vi "get_serv_msgs.vi"() -> ()   [LabVIEW 2010]
uses:
  <vilib>/httpClient/LabVIEWHTTPClient.lvlib
panel:
  out "date/time string":string
  in  "Tab Control":enum32{"Page 1", "Page 2"}(tab)
  out "body":string
  out "Table Control":string[][](table)
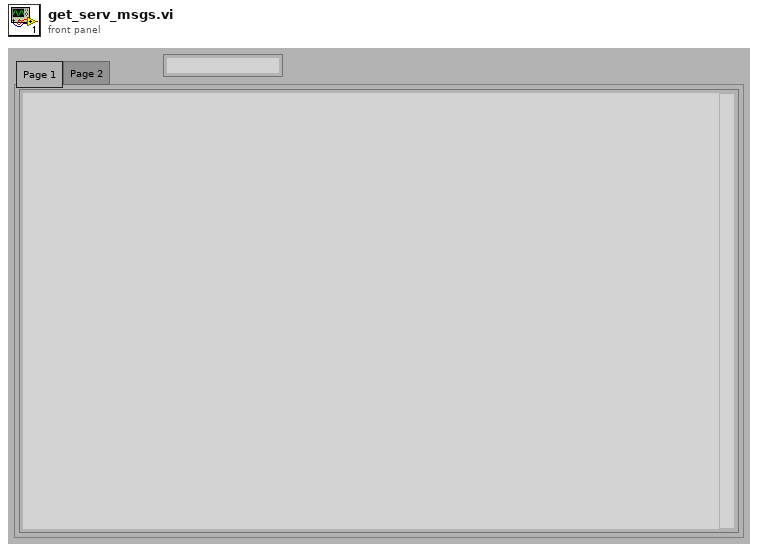
[diagram p1: front panel]
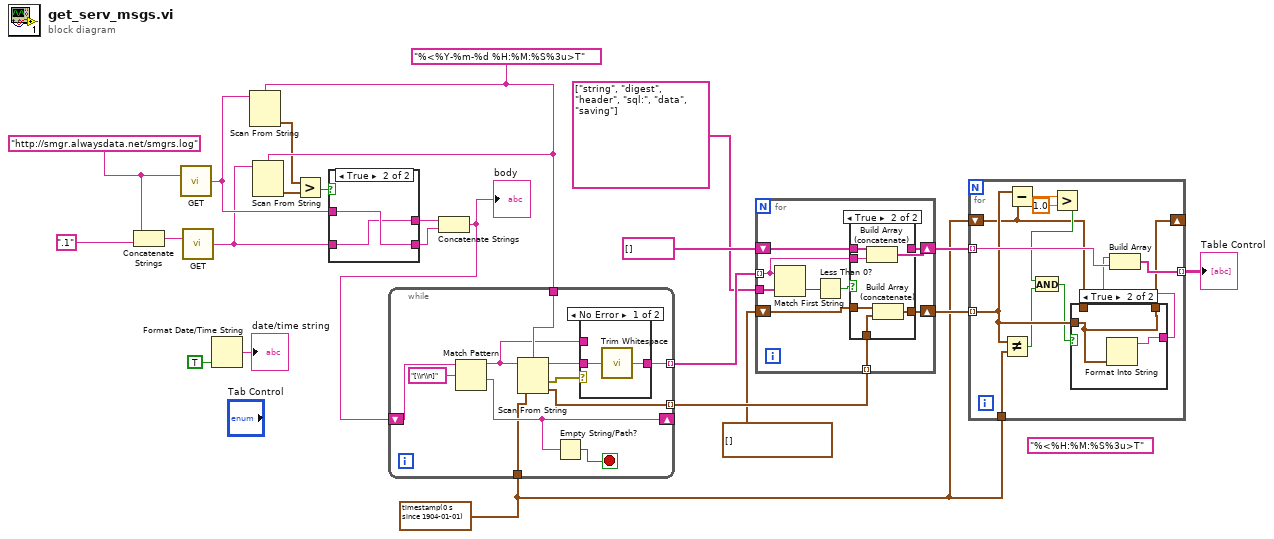
[diagram p0: block diagram]
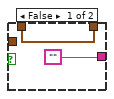
[diagram p2: hidden frame]
diagram:
  (unwired) "%<%H:%M:%S%3u>T" ("format string")
  w3 = timestamp(0 s since 1904-01-01) ("default value 1")
  w15 = "%<%Y-%m-%d %H:%M:%S%3u>T" ("format string")
  w16 = "http://smgr.alwaysdata.net/smgrs.log" ("URL")
  n1 = Concatenate Strings(w16, ".1" ("string")) -> (w19:string)
  n2 = call <vilib>:"GET.vi"("URL"=w16) -> ("body"=w10:string)  [unwired: 11 in, 3 out]
  n3 = call <vilib>:"GET.vi"("URL"=w19) -> ("body"=w9:string)  [unwired: 11 in, 3 out]
  n4 = Format Date/Time String(UTC format=TRUE) -> (date/time string=→"date/time string":string)  [unwired: 2 in]
  n5 = Scan From String(format string=w15, input string=w10) -> (output 1=w14:timestamp)  [unwired: 3 in, 3 out]
  n6 = Scan From String(format string=w15, input string=w9) -> (output 1=w13:timestamp)  [unwired: 3 in, 3 out]
  n7 = Greater?(x=w14, y=w13) -> (0:w12:bool)
  n8 = case shown="True" w12 {
    tunnel: w10 -> [w24 w27]
    tunnel: w9 -> [w25 w26]
    tunnel: [w25 w27] -> w8
    tunnel: [w24 w26] -> w7
    frame False {
    }
    frame True {
    }
  }
  n9 = Concatenate Strings(w7, w8) -> (w11:string)
  "body" <- w11
  n10 = while {
    shift-right: [w35] -> _
    shift-left: w11 -> [w37]
    tunnel: [w31] -> w23 mode=indexing
    tunnel: w15 -> [w34]
    tunnel: [w29] -> w18 mode=indexing
    tunnel: w3 -> [w28]
    stop <- w36 stop-if-true
    n11 = Match Pattern(string=w37, regular expression="[\\r\\n]") -> (before substring=w30:string, after substring=w35:string)  [unwired: 1 in, 2 out]
    n12 = Scan From String(format string=w34, input string=w30, default 1=w28) -> (remaining string=w32:string, error out=w33:errorcluster, output 1=w29:timestamp)  [unwired: 2 in, 1 out]
    n13 = Empty String/Path?(string/path=w35) -> (empty?=w36:bool)
    n14 = case shown="No Error" w33 {
      tunnel: [w39 w41] -> w31
      tunnel: w32 -> [w40 _]
      tunnel: w30 -> [_ w41]
      frame No Error {
        n15 = call <vilib>:"Trim Whitespace.vi"("string"=w40) -> ("trimmed string"=w39:string)  [unwired: 1 in]
      }
      frame Error {
      }
    }
  }
  n16 = for {
    tunnel: w23 -> [w48] mode=indexing
    shift-right: [w47] -> w5
    shift-left: string[] [] -> [w46]
    tunnel: string[] ["string", "digest", "header", "sql:", "data", "saving"] -> [w45]
    tunnel: w18 -> [w44] mode=indexing
    shift-right: [w43] -> w6
    shift-left: timestamp[] [] -> [w42]
    n17 = Match First String(2:w45, 3:w48) -> (0:w50:i32)  [unwired: 1 out]
    n18 = Less Than 0?(x=w50) -> (x < 0?=w49:bool)
    n19 = case shown="True" w49 {
      tunnel: w48 -> [_ w58]
      tunnel: [w52 w57] -> w47
      tunnel: w46 -> [w52 w56]
      tunnel: w44 -> [_ w55]
      tunnel: [w51 w54] -> w43
      tunnel: w42 -> [w51 w53]
      frame False {
      }
      frame True {
        n20 = Build Array (concatenate)(w56, w58) -> (w57:string[])
        n21 = Build Array (concatenate)(w53, w55) -> (w54:timestamp[])
      }
    }
  }
  n22 = for {
    tunnel: w6 -> [w66] mode=indexing
    tunnel: w5 -> [w70] mode=indexing
    tunnel: [w69] -> w4 mode=indexing
    tunnel: w3 -> [w68]
    shift-right: [w60] -> _
    shift-left: w3 -> [w59]
    n23 = Not Equal?(x=w66, y=w68) -> (x != y?=w62:bool)
    n24 = Subtract(x=w66, y=w59) -> (x-y=w65:dbl)
    n25 = Greater?(x=w65, y=1.0) -> (0:w63:bool)
    n26 = And(x=w63, y=w62) -> (x .and. y?=w61:bool)
    n27 = case shown="True" w61 {
      tunnel: ["" w74] -> w67
      tunnel: w66 -> [_ w73]
      tunnel: [w71 w73] -> w60
      tunnel: w59 -> [w71 _]
      frame False {
      }
      frame True {
        n28 = Format Into String(w73) -> (resulting string=w74:string)  [unwired: 3 in, 1 out]
      }
    }
    n29 = Build Array(w67, w70) -> (w69:string[])
  }
  "Table Control" <- w4
